vi "Edit S-parameter data.vi"() -> ()   [LabVIEW 2020]
uses:
  <vilib>/Utility/file.llb/Read Delimited Spreadsheet (string).vi
panel:
  out "all rows":string[][](array[string])
  out "text":string
  in  "file path (use dialog)":path
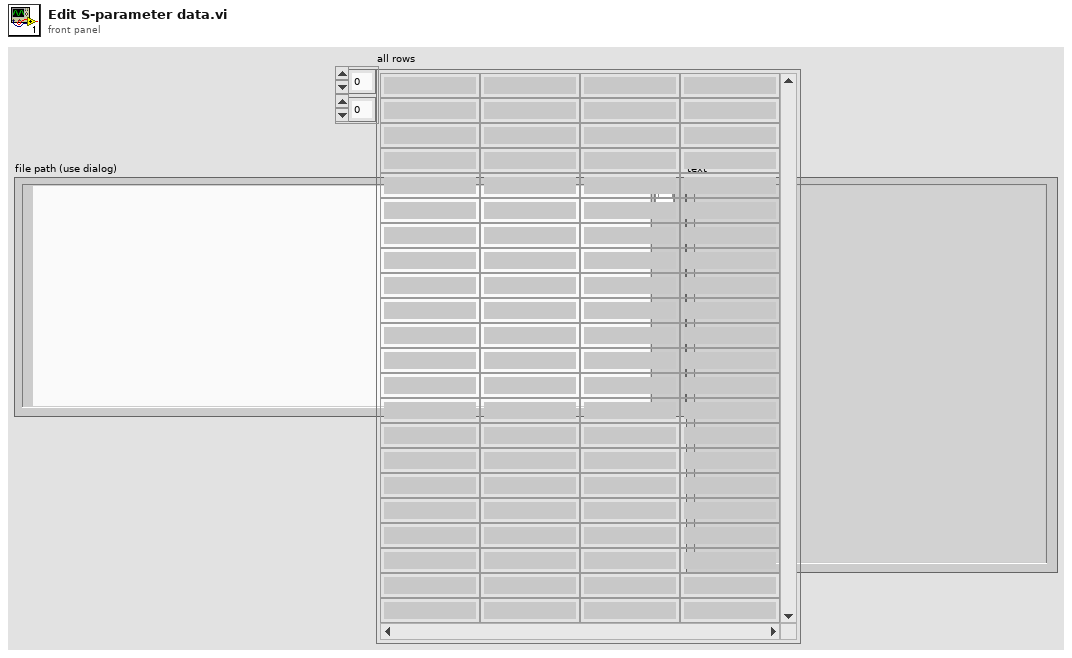
[diagram p1: front panel]
types:
  T1 = enum16{"open", "replace", "create", "open or create", "replace or create", "replace or create with confirmation"}
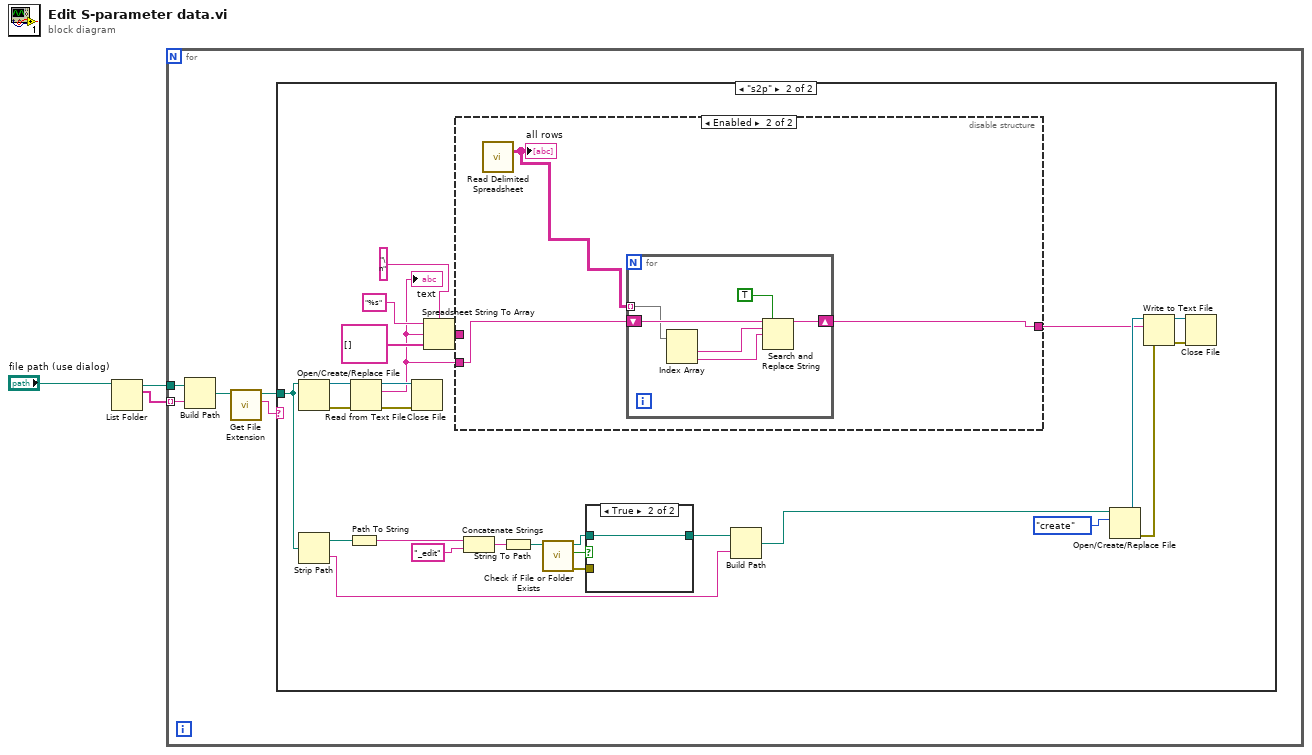
[diagram p0: block diagram]
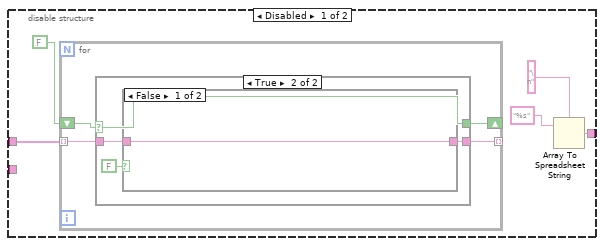
[diagram p3: hidden frame]
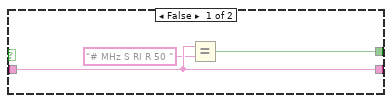
[diagram p4: hidden frame]
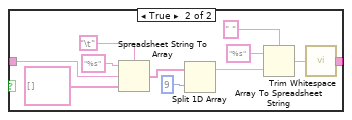
[diagram p5: hidden frame]
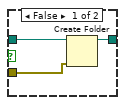
[diagram p6: hidden frame]
diagram:
  n1 = List Folder(path="file path (use dialog)") -> (path out=w2:path, filenames=w1:string[])  [unwired: 3 in, 2 out]
  n2 = for {
    tunnel: w2 -> [w8]
    tunnel: w1 -> [w7] mode=indexing
    n3 = Build Path(base path=w8, name or relative path=w7) -> (appended path=w6:path)
    n4 = call <vilib>:"Get File Extension.vi"("file"=w6) -> ("lowercase file extension"=w4:string, "dup file"=w5:path)  [unwired: 6 in, 3 out]
    n5 = case shown="\"s2p\"" w4 {
      tunnel: w5 -> [_ w11]
      frame Default {
      }
      frame "s2p" {
        n6 = Open/Create/Replace File(file path (use dialog)=w11) -> (refnum out=w35:refnum<file>, error out=w34:errorcluster)  [unwired: 5 in, 1 out]
        n7 = Strip Path(path=w11) -> (stripped path=w27:path, name=w22:string)
        n8 = Path To String(path=w27) -> (string=w26:string)
        n9 = Read from Text File(file (use dialog)=w35, error in=w34) -> (refnum out=w33:refnum<file>, text=w10:string, error out=w32:errorcluster)  [unwired: 2 in, 1 out]
        "text" <- w10
        n10 = Close File(refnum=w33, error in=w32) -> ()  [unwired: 2 out]
        n11 = Spreadsheet String To Array(delimiter (Tab)="\n", format string="%s", spreadsheet string=w10, array type (2D Dbl)=string[] []) -> (array=w28:string[])
        n12 = disable-structure shown="Enabled" {
          disable-tunnel: w28 -> [w42 _]
          disable-tunnel: w10 -> [_ w68]
          disable-tunnel: [w36 w67] -> w9
          frame Disabled {
            n13 = for {
              tunnel: w42 -> [w45] mode=indexing
              tunnel: [w46] -> w40 mode=indexing
              shift-right: [w43] -> _
              shift-left: FALSE -> [w44]
              n14 = case shown="True" w44 {
                selector: w44 -> [_ w53]
                tunnel: [w49 w51] -> w46
                tunnel: w45 -> [w49 w52]
                tunnel: [w47 w53] -> w43
                frame False {
                  n15 = Equal?(x=w49, y="# MHz S RI R 50 ") -> (x = y?=w47:bool)
                }
                frame True {
                  n16 = case shown="False" FALSE {
                    tunnel: w52 -> [w54 w57]
                    tunnel: [w54 w55] -> w51
                    frame False {
                    }
                    frame True {
                      n17 = Spreadsheet String To Array(delimiter (Tab)="\t", format string="%s", spreadsheet string=w57, array type (2D Dbl)=string[] []) -> (array=w60:string[])
                      n18 = Split 1D Array(array=w60, index=9) -> (first subarray=w58:string[])  [unwired: 1 out]
                      n19 = Array To Spreadsheet String(delimiter (Tab)=" ", array=w58, 3:"%s" ("format string")) -> (spreadsheet string=w56:string)
                      n20 = call <vilib>:"Trim Whitespace.vi"("string"=w56) -> ("trimmed string"=w55:string)  [unwired: 1 in]
                    }
                  }
                }
              }
            }
            n21 = Array To Spreadsheet String(delimiter (Tab)="\n", 3:"%s" ("format string")) -> (array=w39:dbl[][], spreadsheet string=w36:string)
          }
          frame Enabled {
            n22 = call-poly <vilib>:"Read Delimited Spreadsheet.vi"() -> ("all rows"=w66:string[][])  [unwired: 10 in, 5 out]
            "all rows" <- w66
            n23 = for {
              shift-right: [w72] -> w67
              shift-left: w68 -> [w74]
              tunnel: w66 -> [w71] mode=indexing
              n24 = Index Array(array=w71) -> (element #1=w70:string, element #2=w69:string)  [unwired: 2 in]
              n25 = Search and Replace String(replace all?=TRUE ("replace all? (F)"), input string=w74, search string=w70, replace string=w69) -> (result string=w72:string)  [unwired: 4 in, 3 out]
            }
          }
        }
        n26 = Concatenate Strings(w26, "_edit" ("string")) -> (w24:string)
        n27 = String To Path(string=w24) -> (path=w15:path)
        n28 = call <vilib>:"Check if File or Folder Exists.vi"("path"=w15) -> ("error out"=w13:errorcluster, "file or folder exists?"=w12:bool, "dup path"=w14:path)  [unwired: 8 in]
        n29 = case shown="True" w12 {
          tunnel: [w77 w78] -> w23
          tunnel: w14 -> [w76 w78]
          tunnel: w13 -> [w75 _]
          frame False {
            n30 = Create Folder(path (use dialog)=w76, error in=w75) -> (created path=w77:path)  [unwired: 1 in, 2 out]
          }
          frame True {
          }
        }
        n31 = Build Path(base path=w23, name or relative path=w22) -> (appended path=w17:path)
        n32 = Open/Create/Replace File(file path (use dialog)=w17, operation (0:open)=T1."create") -> (refnum out=w21:refnum<file>, error out=w20:errorcluster)  [unwired: 4 in, 1 out]
        n33 = Write to Text File(file (use dialog)=w21, text=w9, error in=w20) -> (refnum out=w19:refnum<file>, error out=w18:errorcluster)  [unwired: 1 in, 1 out]
        n34 = Close File(refnum=w19, error in=w18) -> ()  [unwired: 2 out]
      }
    }
  }
